vi "PushToErrorHandler.vi"(7 "MainQ":refnum<queue>, 10 "ErrorIn":errorcluster, 11 "ErrorLocation":string) -> (2 "ErrorOut":errorcluster)   [LabVIEW 2018]
doc: "When <B>ErrorIn</B> contains an error condition, place the error into <B>ClusterIn</B>'s queue member \"Q\".\n\nThe Main (Consumer) Loop dequeues this error and takes appropriate action depending on the error.\n\nCopyright © 2011 Epimedia, Inc. All Rights Reserved.\n\nThe Epimedia Application Library is Copyright © 2009-2011 Epimedia, Inc. \nAll Rights Reserved. Used under license."
uses:
  Queue/RTMainQueueElements.ctl
panel:
  # "Copyright © 2011 Epimedia, Inc. All Rights Reserved.\n\nThe Epimedia Application Library is Copyright © 2009-2011 Epimedia, Inc. \nAll Rights Reserved. Used under license."
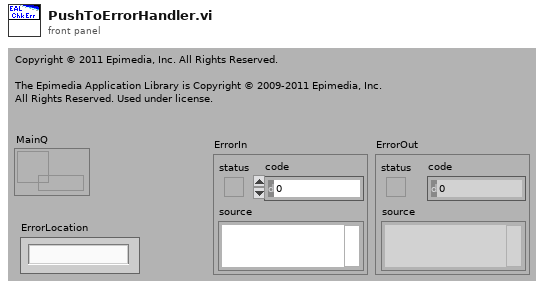
[diagram p1: front panel]
types:
  T1 = typedef "RTMainQueueElements.ctl" = enum16{"RTMain_InitQ", "RTMain_InitSW", "RTMain_InitCtrls", "RTMain_ReInitHW", "RTMain_FromStream", "RTMain_StrtHWLp", "RTMain_UpdtHWClstr", "RTMain_Start", "RTMain_Stop", "RTMain_Error", "RTMain_Config", "RTMain_Exit"}
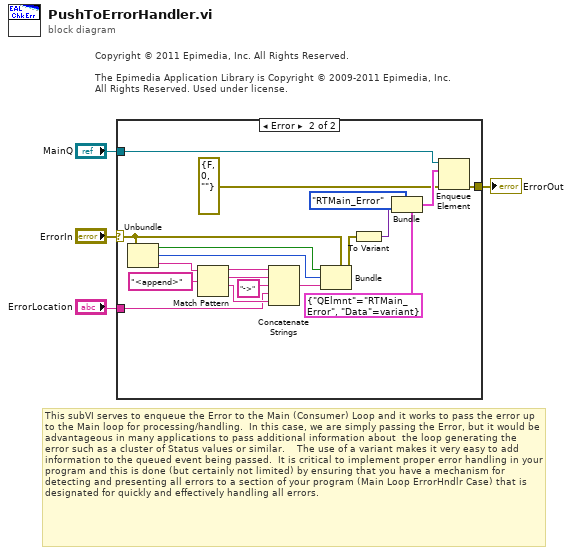
[diagram p0: block diagram]
diagram:
  # "This subVI serves to enqueue the Error to the Main (Consumer) Loop and it works to pass the error up to the Main loop for processing/handling.  In this case, we are simply passing the Error, but it would be advantageous in many applications to pass additional information about  the loop generating the error such as a cluster of Status values or similar.    The use of a variant makes it very easy to add information to the queued event being passed.  It is critical to implement proper error handling in your program and this is done (but certainly not limited) by ensuring that you have a mechanism for detecting and presenting all errors to a section of your program (Main Loop ErrorHndlr Case) that is designated for quickly and effectively handling all errors."
  # "Copyright © 2011 Epimedia, Inc. All Rights Reserved.\n\nThe Epimedia Application Library is Copyright © 2009-2011 Epimedia, Inc. \nAll Rights Reserved. Used under license."
  n1 = case shown="Error" "ErrorIn" {
    selector: "ErrorIn" -> [w5 w8]
    tunnel: [w5 w24] -> w4
    tunnel: "MainQ" -> [_ w18]
    tunnel: "ErrorLocation" -> [_ w9]
    frame No Error {
    }
    frame Error {
      n2 = Unbundle(w8) -> ("status"=w17:bool, "code"=w16:i32, "source"=w6:string)
      n3 = Match Pattern(string=w6, regular expression="<append>") -> (before substring=w14:string, match substring=w13:string, after substring=w12:string)  [unwired: 1 in, 1 out]
      n4 = Concatenate Strings(w14, w13, "->" ("string"), w9, w12) -> (w10:string)
      n5 = Bundle(cluster=w8, "status"=w17, "code"=w16, "source"=w10) -> (w7:errorcluster)
      n6 = To Variant(anything=w7) -> (Variant=w22:variant)
      n7 = Bundle(cluster=cluster{"QElmnt":T1, "Data":variant} {"QElmnt"=enum."RTMain_Error", "Data"=variant} ("Cluster"), "QElmnt"=RTMainQueueElements."RTMain_Error", "Data"=w22) -> (w21:cluster{"QElmnt":T1, "Data":variant})
      n8 = Enqueue Element(queue=w18, element=w21, error in (no error)=errorcluster {"status"=FALSE, "code"=0, "source"=""} ("error IO")) -> (error out=w24:errorcluster)  [unwired: 3 out]
    }
  }
  "ErrorOut" <- w4
